vi "Check critical out of time.vi"(8 "error in (no error)":errorcluster, 11 "Tomo in":refnum<class "Tomo.lvclass">) -> (0 "error out":errorcluster, 3 "Tomo out":refnum<class "Tomo.lvclass">)   [LabVIEW 2012, in "Tomo.lvclass"]
uses:
  Tomo.lvclass
  notice type.ctl
  <vilib>/Distrio/Murmex/GenericMessage/GenericMessage.lvclass
  <vilib>/Distrio/Murmex/Murmex/Murmex.lvclass
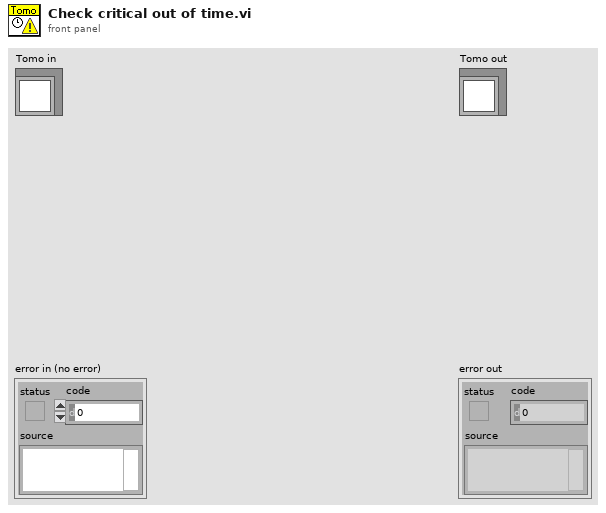
[diagram p1: front panel]
types:
  T1 = typedef "Tomo.lvclass/notice type.ctl" = enum16{"Tomography stopped", "Tomography error", "Tomography finished", "Timing issue", "Critical timing issue"}
  T2 = typedef "Tomo.lvclass/Current activity.ctl" = enum16{"Idle", "Inter-stack motion", "Pre-tomo calculation", "Stack acquisition", "Stack preparation", "Pre-tomo stack acq", "Pre-tomo inter-stack"}
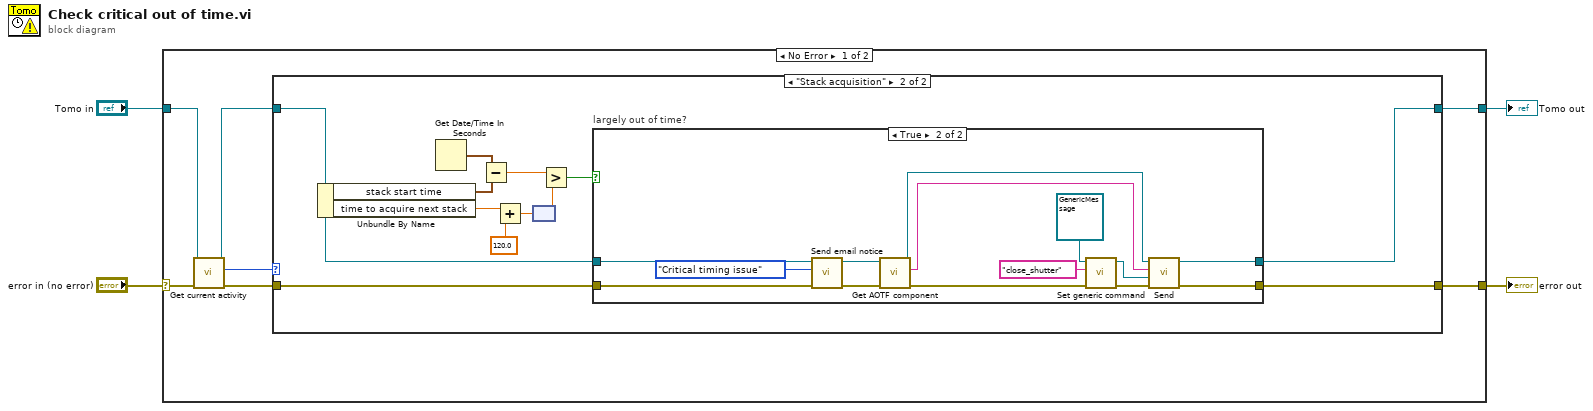
[diagram p0: block diagram]
diagram:
  n1 = case shown="No Error" "error in (no error)" {
    selector: "error in (no error)" -> [w11 w43]
    tunnel: [w7 w43] -> w3
    tunnel: [w5 w42] -> w1
    tunnel: "Tomo in" -> [w10 w42]
    frame No Error {
      n2 = call-dynamic "Get current activity.vi"("error in (no error)"=w11, "Tomo in"=w10) -> ("error out"=w6:errorcluster, "Current activity"=w8:T2, "Tomo out"=w9:refnum<class "Tomo.lvclass">)  [unwired: 7 in]
      n3 = case shown="\"Stack acquisition\"" w8 {
        tunnel: w9 -> [w12 w17]
        tunnel: [w13 w16] -> w7
        tunnel: w6 -> [w13 w18]
        tunnel: [w12 w15] -> w5
        frame "Idle", Default {
        }
        frame "Stack acquisition" {
          n4 = Unbundle By Name(w17) -> ("stack start time"=w24:timestamp, "time to acquire next stack"=w22:dbl[unit])
          n5 = Get Date/Time In Seconds() -> (seconds since 1Jan1904=w25:timestamp)
          n6 = Subtract(x=w25, y=w24) -> (x-y=w23:dbl)
          n7 = Add(x=w22, y=dbl[unit] 120.0) -> (x+y=w20:dbl[unit])
          n8 = node(w20) -> (w19:dbl)
          n9 = Greater?(x=w23, y=w19) -> (0:w14:bool)
          n10 = case "largely out of time?" shown="True" w14 {
            tunnel: w18 -> [w26 w41]
            tunnel: w17 -> [w27 w40]
            tunnel: [w26 w37] -> w16
            tunnel: [w27 w30] -> w15
            frame False {
            }
            frame True {
              n11 = call-dynamic "Send email notice.vi"("error in (no error)"=w41, "Notice type"=notice_type."Critical timing issue", "Tomo in"=w40) -> ("error out"=w36:errorcluster, "Tomo out"=w34:refnum<class "Tomo.lvclass">)  [unwired: 7 in]
              n12 = call-dynamic "Get AOTF component.vi"("error in (no error)"=w36, "Tomo in"=w34) -> ("error out"=w35:errorcluster, "AOTF component"=w28:string, "Tomo out"=w31:refnum<class "Tomo.lvclass">)  [unwired: 7 in]
              n13 = call <vilib>:"Set generic command.vi"("error in (no error)"=w35, "generic command"="close_shutter", "GenericMessage in"=refnum<class "GenericMessage.lvclass"> refnum ("Message in")) -> ("error out"=w38:errorcluster, "GenericMessage out"=w29:refnum<class "GenericMessage.lvclass">)  [unwired: 7 in]
              n14 = call <vilib>:"Send.vi"("error in (no error)"=w38, "Message"=w29, "recipient"=w28, "Murmex in"=w31) -> ("error out"=w37:errorcluster, "Murmex out"=w30:refnum<class "Tomo.lvclass">)  [unwired: 6 in]
            }
          }
        }
      }
    }
    frame Error {
    }
  }
  "error out" <- w3
  "Tomo out" <- w1
